vi "PointAndMotion.vi"(8 "Motion Points":u32, 9 "Motion Increment":u32, 10 "Num Points":u32, 11 "Sample Num":u32) -> (0 "Motion Frame":u32, 1 "Rep Num":u32, 2 "Point Num":u32, 3 "Point Location":u32, 5 "Frame Start":bool)   [LabVIEW 2014]
doc: "Computes the memory location for a given sample number to multiplex between motion tracking and point scanning."
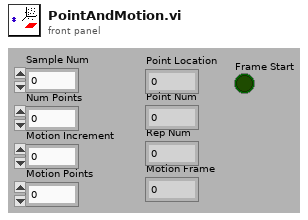
[diagram p1: front panel]
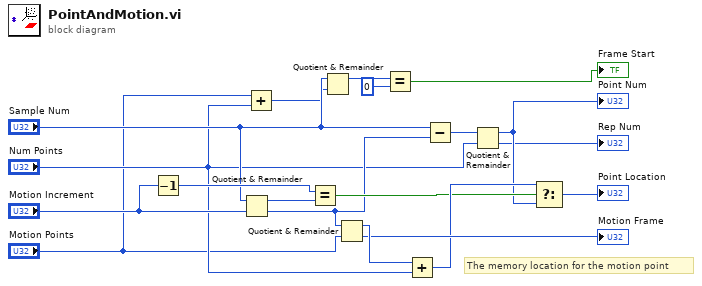
[diagram p0: block diagram]
diagram:
  # "The memory location for the motion point"
  n1 = Decrement(x="Motion Increment") -> (x-1=w9:u32)
  n2 = Quotient & Remainder(x="Sample Num", y="Motion Increment") -> (x-y*floor(x/y)=w19:u32, floor(x/y)=w8:u32)
  n3 = Add(x="Motion Points", y="Num Points") -> (x+y=w6:u32)
  n4 = Equal?(x=w9, y=w19) -> (x = y?=w14:bool)
  n5 = Quotient & Remainder(x="Sample Num", y=w6) -> (x-y*floor(x/y)=w3:u32)  [unwired: 1 out]
  n6 = Quotient & Remainder(x=w8, y="Motion Points") -> (x-y*floor(x/y)=w18:u32, floor(x/y)=→"Motion Frame":u32)
  n7 = Equal?(x=w3, y=u32 0) -> (x = y?=→"Frame Start":bool)
  n8 = Add(x=w18, y="Num Points") -> (x+y=w16:u32)
  n9 = Subtract(x="Sample Num", y=w8) -> (x-y=w15:u32)
  n10 = Quotient & Remainder(x=w15, y="Num Points") -> (x-y*floor(x/y)=w13:u32, floor(x/y)=→"Rep Num":u32)
  "Point Num" <- w13
  n11 = Select(t=w16, s=w14, f=w13) -> (s? t:f=→"Point Location":u32)
